vi "decimate_waveforms.vi"(0 "WFM":waveform(dbl)[](array[waveform]), 1 "averaging":bool, 2 "decimating factor":i32=1, 3 "error in (no error)":errorcluster) -> (7 "WFM out":waveform(dbl)[](array[waveform]), 10 "error out":errorcluster)   [LabVIEW 2016, in "LockinDAQ.lvclass"]
doc: "Decimates the input sequence X by the decimating factor and the averaging Boolean control."
uses:
  LockinDAQ.lvclass
  <vilib>/Analysis/2dsp.llb/Decimate (single shot, DBL).vi
  <vilib>/Analysis/NI_AALPro.lvlib
panel:
  # "by Marco Tedaldi, Brain Research Institute, University of Zurich, 2013"
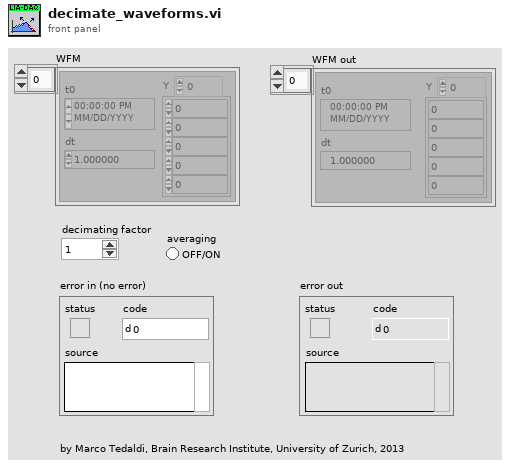
[diagram p1: front panel]
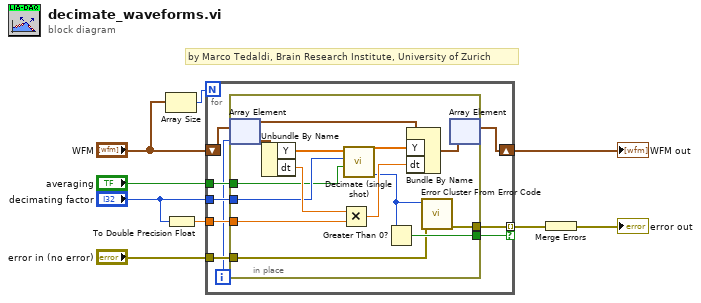
[diagram p0: block diagram]
diagram:
  # "by Marco Tedaldi, Brain Research Institute, University of Zurich"
  n1 = Array Size(array="WFM") -> (size(s)=w5:i32)
  n2 = To Double Precision Float(number="decimating factor") -> (double precision float=w9:dbl)
  n3 = for {
    N: w5 -> [_]
    tunnel: w9 -> [w18]
    tunnel: "decimating factor" -> [w17]
    tunnel: "averaging" -> [w16]
    tunnel: "error in (no error)" -> [w14]
    tunnel: [w13] -> w2 mode=indexing if=w15
    shift-right: [w10] -> w3
    shift-left: "WFM" -> [w12]
    i -> [w11]
    n4 = in-place {
      in-place-border: w18 -> [w28]
      in-place-border: w17 -> [w27]
      in-place-border: w16 -> [w25]
      in-place-border: [w24] -> w15
      in-place-border: w14 -> [w23]
      in-place-border: [w22] -> w13
      n5 = in-place-array #1(w12, w11) -> (w20:waveform(dbl))
      n6 = Unbundle By Name(w20) -> ("Y"=w31:dbl[], "dt"=w29:dbl)
      n7 = Multiply(x=w29, y=w28) -> (x*y=w26:dbl)
      n8 = call-poly <vilib>:"Decimate (single shot).vi"("averaging"=w25, "decimating factor"=w27, "X"=w31) -> ("error"=w21:i32, "Decimated Array"=w30:dbl[])  [unwired: 7 in]
      n9 = Greater Than 0?(x=w21) -> (x > 0?=w24:bool)
      n10 = Bundle By Name(cluster=w20, "Y"=w30, "dt"=w26) -> (w19:waveform(dbl))
      n11 = call <vilib>:"Error Cluster From Error Code.vi"("error in (no error)"=w23, "error code (0)"=w21) -> ("error out"=w22:errorcluster)  [unwired: 7 in]
      n12 = in-place-array #1(w19) -> (w10:waveform(dbl)[])  [unwired: 1 out]
    }
  }
  "WFM out" <- w3
  n13 = Merge Errors(w2) -> (→"error out":errorcluster)
